vi "Reverse 2D Array__ogtk.vi"   [LabVIEW 2016]
doc: "This polymorphic VI reverses the input 2D <B>Array</B> and outputs the result as <B>Reversed Array</B>. Use the <B>by rows or columns</B> input to specify whether to sort by row or by column."
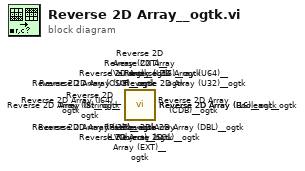
[diagram p0: block diagram]
diagram:
  n1 = call <userlib>:"Reverse 2D Array (LVObject)__ogtk.vi"() -> ()  [unwired: 3 in, 1 out]
  n2 = call <userlib>:"Reverse 2D Array (U64)__ogtk.vi"() -> ()  [unwired: 3 in, 1 out]
  n3 = call <userlib>:"Reverse 2D Array (I64)__ogtk.vi"() -> ()  [unwired: 3 in, 1 out]
  n4 = call <userlib>:"Reverse 2D Array (CDB)__ogtk.vi"() -> ()  [unwired: 3 in, 1 out]
  n5 = call <userlib>:"Reverse 2D Array (CSG)__ogtk.vi"() -> ()  [unwired: 3 in, 1 out]
  n6 = call <userlib>:"Reverse 2D Array (CXT)__ogtk.vi"() -> ()  [unwired: 3 in, 1 out]
  n7 = call <userlib>:"Reverse 2D Array (DBL)__ogtk.vi"() -> ()  [unwired: 3 in, 1 out]
  n8 = call <userlib>:"Reverse 2D Array (EXT)__ogtk.vi"() -> ()  [unwired: 3 in, 1 out]
  n9 = call <userlib>:"Reverse 2D Array (I16)__ogtk.vi"() -> ()  [unwired: 3 in, 1 out]
  n10 = call <userlib>:"Reverse 2D Array (I32)__ogtk.vi"() -> ()  [unwired: 3 in, 1 out]
  n11 = call <userlib>:"Reverse 2D Array (I8)__ogtk.vi"() -> ()  [unwired: 3 in, 1 out]
  n12 = call <userlib>:"Reverse 2D Array (SGL)__ogtk.vi"() -> ()  [unwired: 3 in, 1 out]
  n13 = call <userlib>:"Reverse 2D Array (U16)__ogtk.vi"() -> ()  [unwired: 3 in, 1 out]
  n14 = call <userlib>:"Reverse 2D Array (U32)__ogtk.vi"() -> ()  [unwired: 3 in, 1 out]
  n15 = call <userlib>:"Reverse 2D Array (U8)__ogtk.vi"() -> ()  [unwired: 3 in, 1 out]
  n16 = call <userlib>:"Reverse 2D Array (Boolean)__ogtk.vi"() -> ()  [unwired: 3 in, 1 out]
  n17 = call <userlib>:"Reverse 2D Array (String)__ogtk.vi"() -> ()  [unwired: 3 in, 1 out]
  n18 = call <userlib>:"Reverse 2D Array (Path)__ogtk.vi"() -> ()  [unwired: 3 in, 1 out]
  n19 = call <userlib>:"Reverse 2D Array (Variant)__ogtk.vi"() -> ()  [unwired: 3 in, 1 out]
